vi "lab2.vi"() -> ()   [LabVIEW 2020]
panel:
  out "time":dbl
  out "Boolean 8":bool
  out "Boolean 7":bool
  out "Boolean 6":bool
  out "Boolean 5":bool
  out "Boolean 4":bool
  out "Boolean 3":bool
  out "Boolean 2":bool
  out "Boolean":bool
  out "S":dbl
  in  "e":dbl
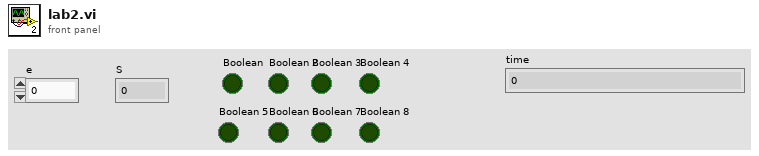
[diagram p1: front panel]
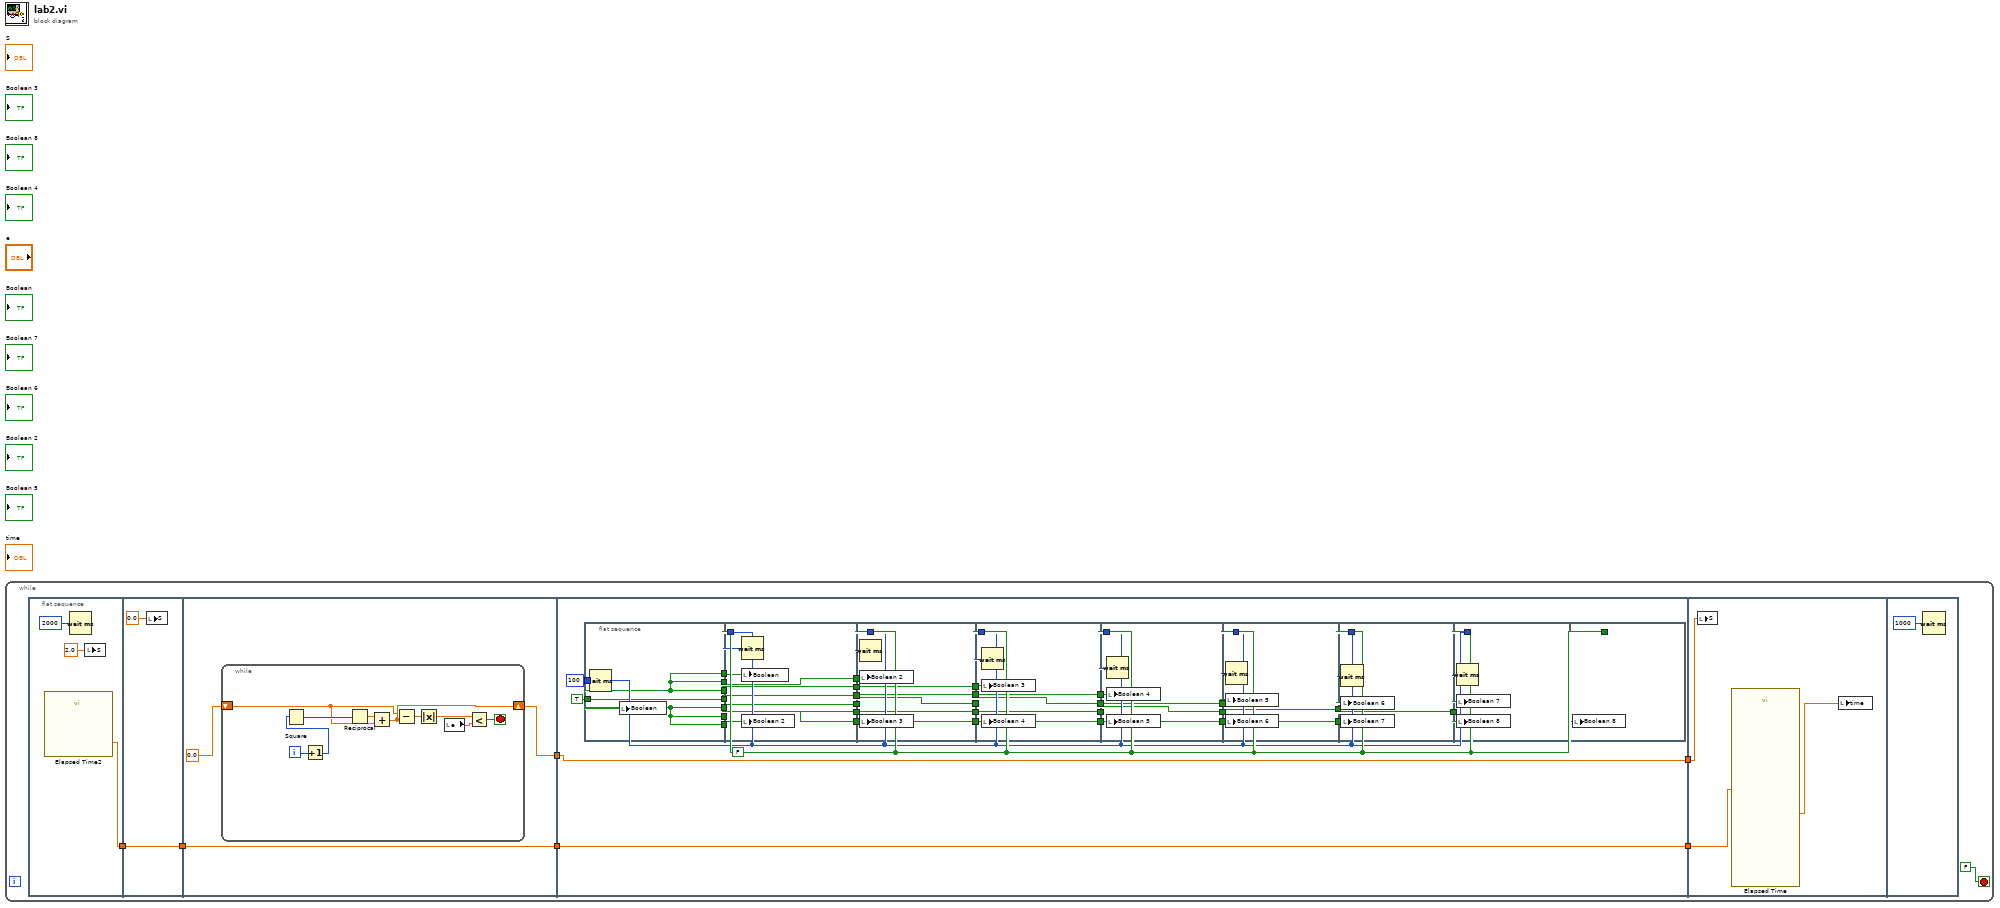
[diagram p0: block diagram]
diagram:
  n1 = while {
    stop <- FALSE stop-if-true
    n2 = flat-sequence {
      tunnel: [w8] -> w1
      tunnel: [w11] -> w2
      tunnel: w1 -> [w11]
      tunnel: [w15] -> w7
      tunnel: [w13] -> w3
      tunnel: w2 -> [w13]
      tunnel: w7 -> [w58]
      tunnel: [w58] -> w6
      tunnel: [w26] -> w4
      tunnel: w3 -> [w26]
      tunnel: w6 -> [w106]
      tunnel: w4 -> [w104]
      frame #0 {
        n3 = call "Elapsed Time2"() -> ("Get Start Time (s)"=w8:dbl)  [unwired: 12 in, 7 out]
        n4 = Wait (ms)(milliseconds to wait=u32 2000) -> ()  [unwired: 1 out]
        n5 = local write "S"(2.0 ("S")) -> ()
      }
      frame #1 {
        n6 = local write "S"(0.0 ("S")) -> ()
      }
      frame #2 {
        n7 = while {
          shift-right: [w21] -> w15
          shift-left: 0.0 -> [w20]
          i -> [w25]
          stop <- w16 stop-if-true
          n8 = Increment(x=w25) -> (x+1=w24:i32)
          n9 = Square(x=w24) -> (x^2=w23:i32)
          n10 = Reciprocal(x=w23) -> (1/x=w22:dbl)
          n11 = Add(x=w22, y=w20) -> (x+y=w21:dbl)
          n12 = Subtract(x=w20, y=w21) -> (x-y=w19:dbl)
          n13 = Absolute Value(x=w19) -> (abs(x)=w18:dbl)
          n14 = local read "e"() -> (w17:dbl)
          n15 = Less?(x=w18, y=w17) -> (x < y?=w16:bool)
        }
      }
      frame #3 {
        w27 = u32 100 ("milliseconds to wait")
        w28 = FALSE
        n16 = flat-sequence {
          tunnel: TRUE -> [w60]
          tunnel: [w60] -> w56
          tunnel: [w60] -> w55
          tunnel: [w60] -> w53
          tunnel: [w60] -> w50
          tunnel: [w60] -> w46
          tunnel: [w60] -> w41
          tunnel: [w60] -> w35
          tunnel: w27 -> [w59]
          tunnel: w56 -> [w69]
          tunnel: w55 -> [w68]
          tunnel: [w68] -> w54
          tunnel: w53 -> [w67]
          tunnel: [w67] -> w52
          tunnel: w50 -> [w66]
          tunnel: [w66] -> w49
          tunnel: w46 -> [w65]
          tunnel: [w65] -> w45
          tunnel: w41 -> [w64]
          tunnel: [w64] -> w40
          tunnel: w35 -> [w63]
          tunnel: [w63] -> w34
          tunnel: w28 -> [w62]
          tunnel: w27 -> [w61]
          tunnel: w54 -> [w77]
          tunnel: w52 -> [w76]
          tunnel: [w76] -> w51
          tunnel: w49 -> [w75]
          tunnel: [w75] -> w48
          tunnel: w45 -> [w74]
          tunnel: [w74] -> w44
          tunnel: w40 -> [w73]
          tunnel: [w73] -> w39
          tunnel: w34 -> [w72]
          tunnel: [w72] -> w33
          tunnel: w28 -> [w71]
          tunnel: w27 -> [w70]
          tunnel: w51 -> [w84]
          tunnel: w48 -> [w83]
          tunnel: [w83] -> w47
          tunnel: w44 -> [w82]
          tunnel: [w82] -> w43
          tunnel: w39 -> [w81]
          tunnel: [w81] -> w38
          tunnel: w33 -> [w80]
          tunnel: [w80] -> w32
          tunnel: w28 -> [w79]
          tunnel: w27 -> [w78]
          tunnel: w47 -> [w90]
          tunnel: w43 -> [w89]
          tunnel: [w89] -> w42
          tunnel: w38 -> [w88]
          tunnel: [w88] -> w37
          tunnel: w32 -> [w87]
          tunnel: [w87] -> w31
          tunnel: w28 -> [w86]
          tunnel: w27 -> [w85]
          tunnel: w42 -> [w95]
          tunnel: w37 -> [w94]
          tunnel: [w94] -> w36
          tunnel: w31 -> [w93]
          tunnel: [w93] -> w30
          tunnel: w28 -> [w92]
          tunnel: w27 -> [w91]
          tunnel: w36 -> [w99]
          tunnel: w30 -> [w98]
          tunnel: [w98] -> w29
          tunnel: w28 -> [w97]
          tunnel: w27 -> [w96]
          tunnel: w29 -> [w102]
          tunnel: w28 -> [w101]
          tunnel: w27 -> [w100]
          tunnel: w28 -> [w103]
          frame #0 {
            n17 = Wait (ms)(milliseconds to wait=w59) -> ()  [unwired: 1 out]
            n18 = local write "Boolean"(w60) -> ()
          }
          frame #1 {
            n19 = Wait (ms)(milliseconds to wait=w61) -> ()  [unwired: 1 out]
            n20 = local write "Boolean"(w62) -> ()
            n21 = local write "Boolean 2"(w69) -> ()
          }
          frame #2 {
            n22 = Wait (ms)(milliseconds to wait=w70) -> ()  [unwired: 1 out]
            n23 = local write "Boolean 2"(w71) -> ()
            n24 = local write "Boolean 3"(w77) -> ()
          }
          frame #3 {
            n25 = Wait (ms)(milliseconds to wait=w78) -> ()  [unwired: 1 out]
            n26 = local write "Boolean 3"(w79) -> ()
            n27 = local write "Boolean 4"(w84) -> ()
          }
          frame #4 {
            n28 = Wait (ms)(milliseconds to wait=w85) -> ()  [unwired: 1 out]
            n29 = local write "Boolean 4"(w86) -> ()
            n30 = local write "Boolean 5"(w90) -> ()
          }
          frame #5 {
            n31 = Wait (ms)(milliseconds to wait=w91) -> ()  [unwired: 1 out]
            n32 = local write "Boolean 5"(w92) -> ()
            n33 = local write "Boolean 6"(w95) -> ()
          }
          frame #6 {
            n34 = Wait (ms)(milliseconds to wait=w96) -> ()  [unwired: 1 out]
            n35 = local write "Boolean 6"(w97) -> ()
            n36 = local write "Boolean 7"(w99) -> ()
          }
          frame #7 {
            n37 = Wait (ms)(milliseconds to wait=w100) -> ()  [unwired: 1 out]
            n38 = local write "Boolean 7"(w101) -> ()
            n39 = local write "Boolean 8"(w102) -> ()
          }
          frame #8 {
            n40 = local write "Boolean 8"(w103) -> ()
          }
        }
      }
      frame #4 {
        n41 = local write "S"(w106) -> ()
        n42 = call "Elapsed Time"("Set Start Time (s)"=w104) -> ("Elapsed Time (s)"=w105:dbl)  [unwired: 11 in, 7 out]
        n43 = local write "time"(w105) -> ()
      }
      frame #5 {
        n44 = Wait (ms)(milliseconds to wait=u32 1000) -> ()  [unwired: 1 out]
      }
    }
  }
